vi "FIR_filter.vi"() -> ()   [LabVIEW 2017]
uses:
  <vilib>/sound2/lvsound2.llb/Sound Data Format.ctl
  <vilib>/Utility/file.llb/Read Delimited Spreadsheet (DBL).vi
  <vilib>/sound2/lvsound2.llb/Sound File Info (path).vi
panel:
  out "coefficients reader":dbl[](array[numeric])
  out "S/s":dbl
  out "s/S":dbl
  out "Signal Output":waveform(dbl)(graph)
  out "FFT Output":cluster{"f0":dbl, "df":dbl, "magnitude":dbl[]}(graph)
  out "Signal Output":waveform(dbl)(graph)
  out "FFT Input":cluster{"f0":dbl, "df":dbl, "magnitude":dbl[]}(graph)
  out "sound format":T1={"sample rate (S/s)"=22050.0, "number of channels"=2, "bits per sample"=16}
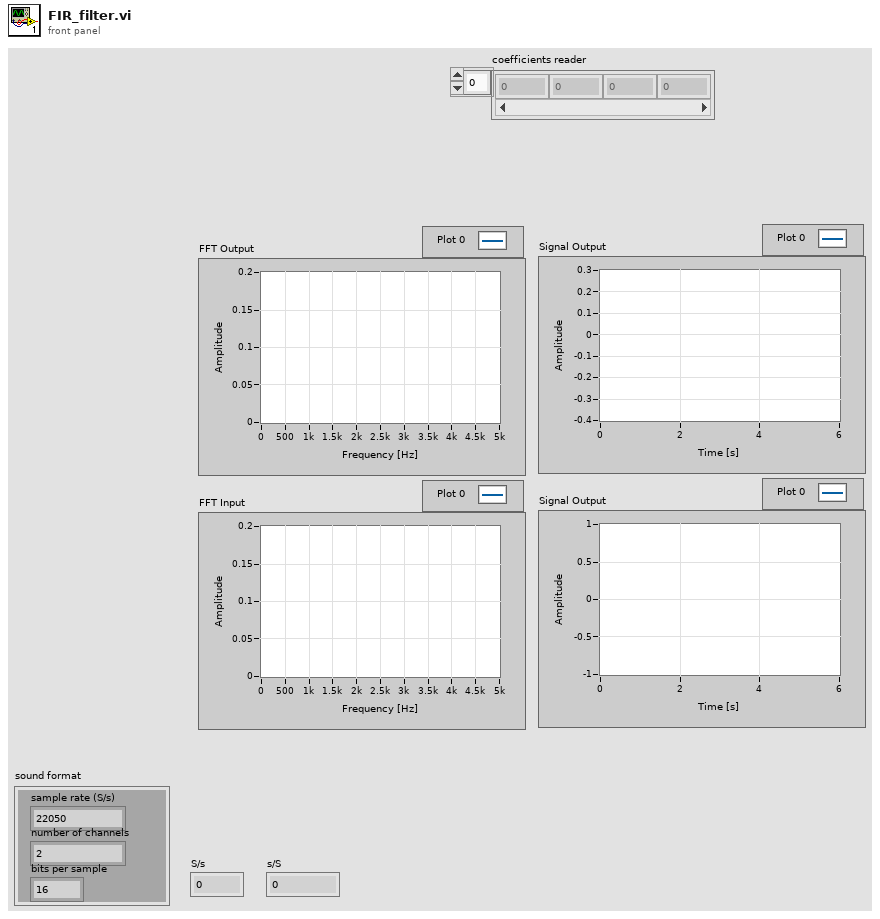
[diagram p1: front panel]
types:
  T1 = typedef "Sound Data Format.ctl" = cluster{"sample rate (S/s)":dbl, "number of channels":i32, "bits per sample":i32}
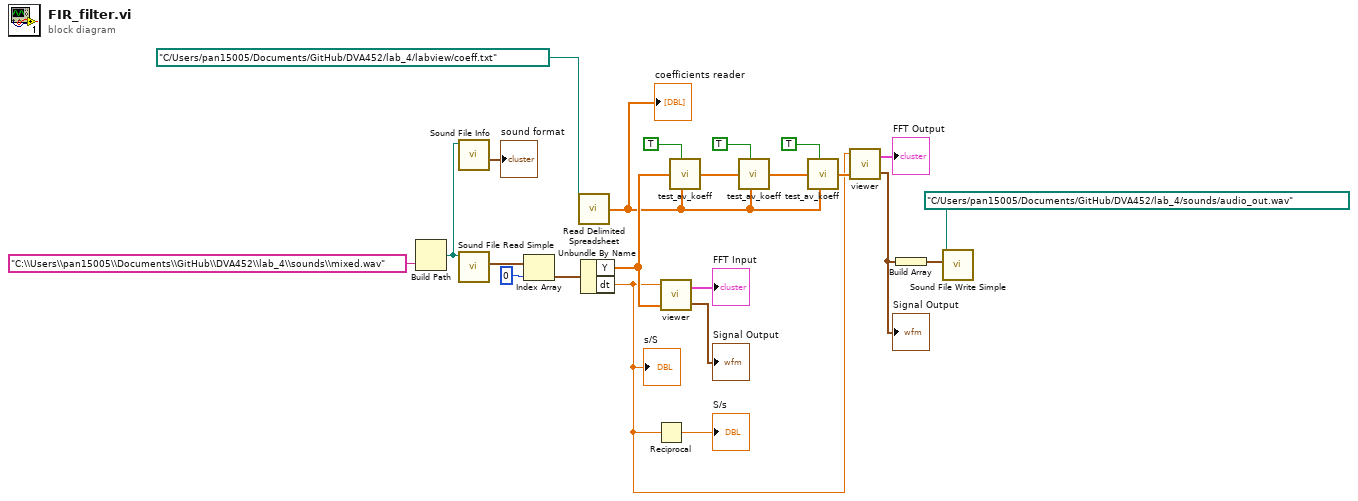
[diagram p0: block diagram]
diagram:
  n1 = Build Path(name or relative path="C:\\Users\\pan15005\\Documents\\GitHub\\DVA452\\lab_4\\sounds\\mixed.wav") -> (appended path=w19:path)  [unwired: 1 in]
  n2 = call-poly <vilib>:"Sound File Info.vi"("path"=w19) -> ("sound format"=→"sound format":T1)  [unwired: 7 in, 3 out]
  n3 = call <vilib>:"Sound File Read Simple.vi"("path"=w19) -> ("data"=w23:waveform(dbl)[])  [unwired: 7 in, 3 out]
  n4 = Index Array(array=w23, index=0) -> (element=w21:waveform(dbl))
  n5 = call-poly <vilib>:"Read Delimited Spreadsheet.vi"("file path (dialog if empty)"=path "C:/Users/pan15005/Documents/GitHub/DVA452/lab_4/labview/coeff.txt") -> ("first row"=w6:dbl[])  [unwired: 9 in, 5 out]
  "coefficients reader" <- w6
  n6 = Unbundle By Name(w21) -> ("Y"=w9:dbl[], "dt"=w4:dbl)
  "s/S" <- w4
  n7 = Reciprocal(x=w4) -> (1/x=→"S/s":dbl)
  n8 = call "viewer.vi"("in"=w9, "f_s"=w4) -> ("Time-Domain"=→"Signal Output":waveform(dbl), "Spectrum"=→"FFT Input":cluster{"f0":dbl, "df":dbl, "magnitude":dbl[]})  [unwired: 1 in]
  n9 = call "test_av_koeff.vi"("s"=TRUE, "in"=w9, "FIR Coefficients"=w6) -> ("out"=w5:dbl[])  [unwired: 4 in]
  n10 = call "test_av_koeff.vi"("s"=TRUE ("enable"), "in"=w5, "FIR Coefficients"=w6) -> ("out"=w11:dbl[])  [unwired: 4 in]
  n11 = call "test_av_koeff.vi"("s"=TRUE, "in"=w11, "FIR Coefficients"=w6) -> ("out"=w10:dbl[])  [unwired: 4 in]
  n12 = call "viewer.vi"("in"=w10, "f_s"=w4) -> ("Time-Domain"=w13:waveform(dbl), "Spectrum"=→"FFT Output":cluster{"f0":dbl, "df":dbl, "magnitude":dbl[]})  [unwired: 1 in]
  "Signal Output" <- w13
  n13 = Build Array(w13) -> (w14:waveform(dbl)[])
  n14 = call <vilib>:"Sound File Write Simple.vi"("data"=w14, "path"=path "C:/Users/pan15005/Documents/GitHub/DVA452/lab_4/sounds/audio_out.wav") -> ()  [unwired: 8 in, 2 out]
